vi "TestInitializeTriggeredSubscription_RejectOldValue.vi"(8 "error in (no error)":errorcluster, 11 "TestCase in":refnum<class "TestSubscriptionPolicy.lvclass">) -> (0 "error out":errorcluster, 3 "TestCase out":refnum<class "TestSubscriptionPolicy.lvclass">)   [LabVIEW 2015, in "TestSubscriptionPolicy.lvclass"]
uses:
  TestSubscriptionPolicy.lvclass
  Framework/SubscriptionPolicy/TriggeredSubscription/Trigger Condition.ctl
  Framework/SubscriptionPolicy/TriggeredSubscription/TriggeredSubscription.lvclass/TriggeredSubscription.ctl
  Framework/SubscriptionPolicy/TriggeredSubscription/TriggeredSubscription.lvclass
  Framework/Transport/QueueTransport/QueueTransport.lvclass
  Framework/IMediator/ISubscriptionPolicy/ISubscriptionPolicy.lvclass
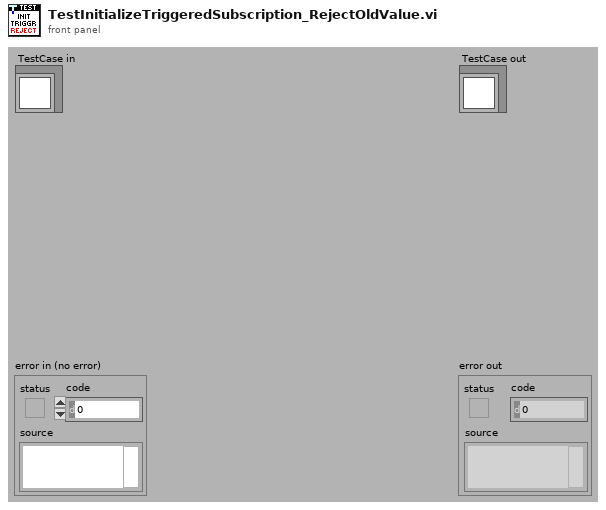
[diagram p1: front panel]
types:
  T1 = typedef "SubscriptionPolicy.lvlib/TriggeredSubscription.lvclass/Trigger Condition.ctl" = enum16{"Equal", "Not equal", "Greater than", "Less than", "Greater or equal", "Less or equal"}
  T2 = cluster{"Data":variant, "Publication Time":timestamp}
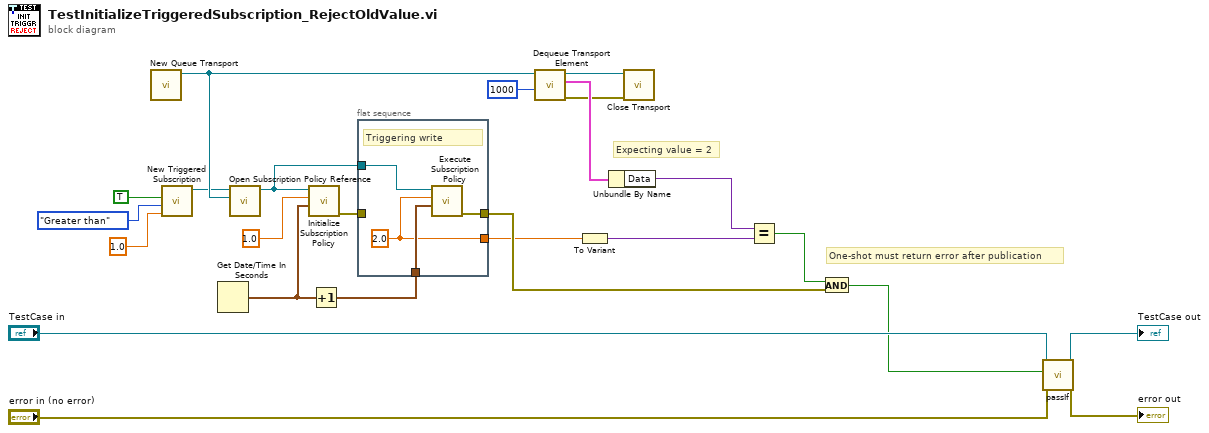
[diagram p0: block diagram]
diagram:
  # "One-shot must return error after publication"
  # "Expecting value = 2"
  n1 = call "New Queue Transport.vi"() -> ("QueueTransport Out"=w20:refnum<class "QueueTransport.lvclass">)  [unwired: 10 in, 1 out]
  n2 = call "New Triggered Subscription.vi"("Trigger Value"=1.0, "Trigger Condition"=Trigger_Condition."Greater than", "Ignore Past Updates? (F)"=TRUE) -> ("OneShotSubscription Out"=w15:refnum<class "TriggeredSubscription.lvclass">)  [unwired: 8 in]
  n3 = Get Date/Time In Seconds() -> (seconds since 1Jan1904=w5:timestamp)
  n4 = call "Open Subscription Policy Reference.vi"("Transport"=w20, "SubscriptionPolicy"=w15) -> ("Subscription Policy"=w6:refnum<data-value>)  [unwired: 8 in, 1 out]
  n5 = call "Initialize Subscription Policy.vi"("Last Publish Time"=w5, "Last Topic Value"=1.0, "Subscription Policy"=w6) -> ("Error Out (Do Not Subscribe?)"=w1:errorcluster)  [unwired: 8 in]
  n6 = Increment(x=w5) -> (x+1=w4:timestamp)
  n7 = flat-sequence {
    tunnel: w6 -> [w28]
    tunnel: w4 -> [w27]
    tunnel: [w26] -> w3
    tunnel: [w25] -> w2
    tunnel: w1 -> [_]
    frame #0 {
      w25 = 2.0
      # "Triggering write"
      n8 = call "Execute Subscription Policy.vi"("Publish Time"=w27, "New Topic Value"=w25, "Subscription Policy"=w28) -> ("error out (Unsubscribe?)"=w26:errorcluster)  [unwired: 8 in]
    }
  }
  n9 = call "Dequeue Transport Element.vi"("Timeout In ms (-1)"=1000, "QueueTransport in"=w20) -> ("error out"=w16:errorcluster, "Element"=w18:T2, "QueueTransport out"=w17:refnum<class "QueueTransport.lvclass">)  [unwired: 6 in, 1 out]
  n10 = To Variant(anything=w2) -> (Variant=w11:variant)
  n11 = Unbundle By Name(w18) -> ("Data"=w13:variant)
  n12 = call-dynamic "Close Transport.vi"("error in (no error)"=w16, "QueueTransport in"=w17) -> ()  [unwired: 9 in, 1 out]
  n13 = Equal?(x=w13, y=w11) -> (x = y?=w10:bool)
  n14 = And(x=w10, y=w3) -> (x .and. y?=w9:bool)
  n15 = call-dynamic "passIf.vi"("error in (no error)"="error in (no error)", "pass"=w9, "TestCase in"="TestCase in") -> ("error out"=→"error out":errorcluster, "TestCase out"=→"TestCase out":refnum<class "TestSubscriptionPolicy.lvclass">)  [unwired: 7 in]
